vi "rapid_xy.vi"(11 "Channel A Out":dbl[][][](array[numeric])) -> (3 "xy array":T1(array[cluster]))   [LabVIEW 2016]
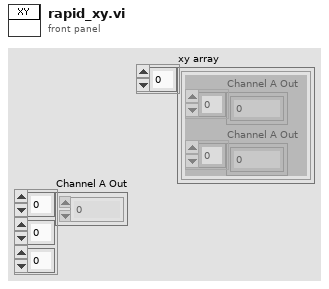
[diagram p1: front panel]
types:
  T1 = cluster{"Channel A Out":dbl[], "Channel A Out":dbl[]}[]
  T2 = cluster{"Channel A Out":dbl[], "Channel A Out":dbl[]}
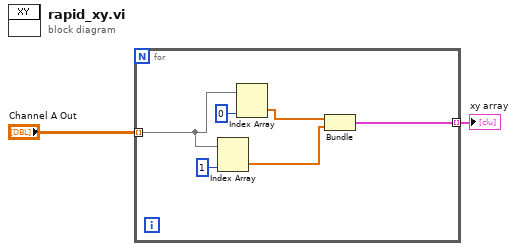
[diagram p0: block diagram]
diagram:
  n1 = for {
    tunnel: "Channel A Out" -> [w4] mode=indexing
    tunnel: [w3] -> w1 mode=indexing
    n2 = Index Array(array=w4, index (col)=1 ("disabled index (col)")) -> (element=w5:dbl[])  [unwired: 1 in]
    n3 = Index Array(array=w4, index (col)=0 ("disabled index (col)")) -> (element=w6:dbl[])  [unwired: 1 in]
    n4 = Bundle("Channel A Out"=w6, "Channel A Out"=w5) -> (w3:T2)  [unwired: 1 in]
  }
  "xy array" <- w1
